vi "Read Trace.vi"(8 "error in (no error)":errorcluster, 9 "Maximum Time (10000)":u32=10000, 11 "VISA resource name":refnum<visa-resource-name>) -> (0 "error out":errorcluster, 2 "Trace Waveform":T1(graph), 3 "VISA resource name out":refnum<visa-resource-name>)   [LabVIEW 2013, in "Template - Spectrum Analyzer.lvlib"]
doc: "Reads a trace from the spectrum analyzer."
uses:
  <instrlib>/_Template - Spectrum Analyzer/Template - Spectrum Analyzer.lvlib
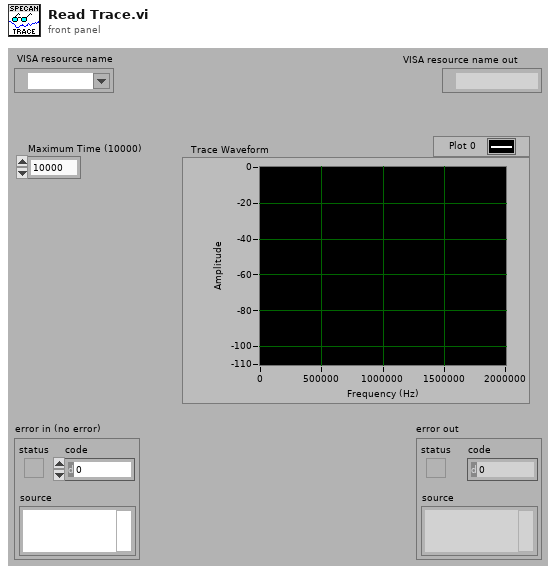
[diagram p1: front panel]
types:
  T1 = cluster{"Start Frequency (0 Hz)":dbl, dbl, "Trace":sgl[]}
  T2 = cluster{"Initial X":dbl, "X Increment":dbl, "Trace Array":sgl[]}
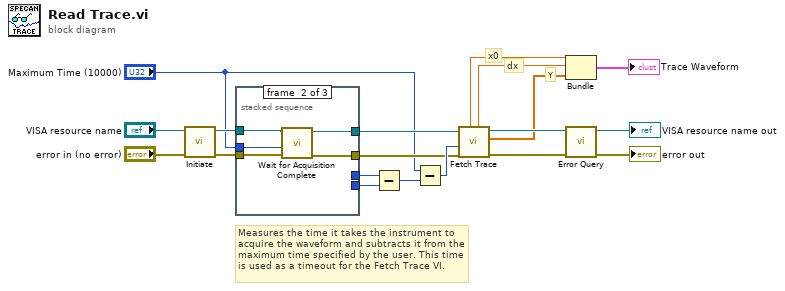
[diagram p0: block diagram]
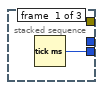
[diagram p2: hidden frame]
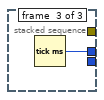
[diagram p3: hidden frame]
diagram:
  # "Measures the time it takes the instrument to acquire the waveform and subtracts it from the maximum time specified by the user. This time is used as a timeout for the Fetch Trace VI."
  # "Y"
  # "dx"
  # "x0"
  n1 = call <instrlib>:"Initiate.vi"("error in (no error)"="error in (no error)", "VISA resource name"="VISA resource name") -> ("error out"=w3:errorcluster, "VISA resource name out"=w5:refnum<visa-resource-name>)  [unwired: 8 in]
  n2 = stacked-sequence {
    tunnel: [w20 _ _] -> w8
    tunnel: [_ _ w26] -> w7
    tunnel: w5 -> [_ w25 _]
    tunnel: [_ w24 _] -> w4
    tunnel: w3 -> [_ w23 _]
    tunnel: [_ w22 _] -> w2
    tunnel: "Maximum Time (10000)" -> [_ w21 _]
    frame #0 {
      n3 = Tick Count (ms)() -> (millisecond timer value=w20:u32)
    }
    frame #1 {
      n4 = call <instrlib>:"Wait for Acquisition Complete.vi"("error in (no error)"=w23, "Maximum Time (10000)"=w21, "VISA resource name"=w25) -> ("error out"=w22:errorcluster, "VISA resource name out"=w24:refnum<visa-resource-name>)  [unwired: 7 in]
    }
    frame #2 {
      n5 = Tick Count (ms)() -> (millisecond timer value=w26:u32)
    }
  }
  n6 = Subtract(x=w7, y=w8) -> (x-y=w9:u32)
  n7 = Subtract(x="Maximum Time (10000)", y=w9) -> (x-y=w6:u32)
  n8 = call <instrlib>:"Fetch Trace.vi"("error in (no error)"=w2, "Timeout (10000 ms)"=w6, "VISA resource name"=w4) -> ("error out"=w15:errorcluster, "Trace Array"=w10:sgl[], "VISA resource name out"=w17:refnum<visa-resource-name>, "X Increment"=w13:dbl, "Initial X"=w12:dbl)  [unwired: 4 in]
  n9 = Bundle("Initial X"=w12, "X Increment"=w13, "Trace Array"=w10) -> (→"Trace Waveform":T2)  [unwired: 1 in]
  n10 = call <instrlib>:"Error Query.vi"("error in (no error)"=w15, "VISA resource name"=w17) -> ("error out"=→"error out":errorcluster, "VISA resource name out"=→"VISA resource name out":refnum<visa-resource-name>)  [unwired: 6 in, 2 out]
